vi "R1NH4Control.vi"(8 "error constant":errorcluster, 11 "LabVIEW Web Service":refnum<class "Web Service.lvclass">) -> (0 "error (out)":errorcluster)   [LabVIEW 2016]
uses:
  <vilib>/wsapi/Web Service.lvclass
  Controls/Tri State Control.ctl
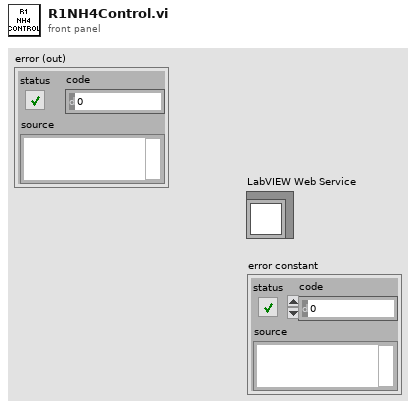
[diagram p1: front panel]
types:
  T1 = cluster{"Signal, mA":dbl, "Value, UNITS HERE":dbl}
  T2 = cluster{"Media Pump":bool, "Water Pump":bool, "Effluent Pump":bool, "Release Valve":bool, "Gas Pump":bool}
  T3 = cluster{"Set Point, mgN/L":dbl, "Tolerance, mgN/L":dbl, "Pump Gain":dbl, "Max Volume/Cycle, mL":dbl}
  T4 = typedef "Tri State Control.ctl" = u16
  T5 = cluster{"Raw Value":dbl, "Corrected Value":dbl, "Signal, mV":dbl, "Equilibrium Approach, mV/min":dbl, "Steady State?":T4}
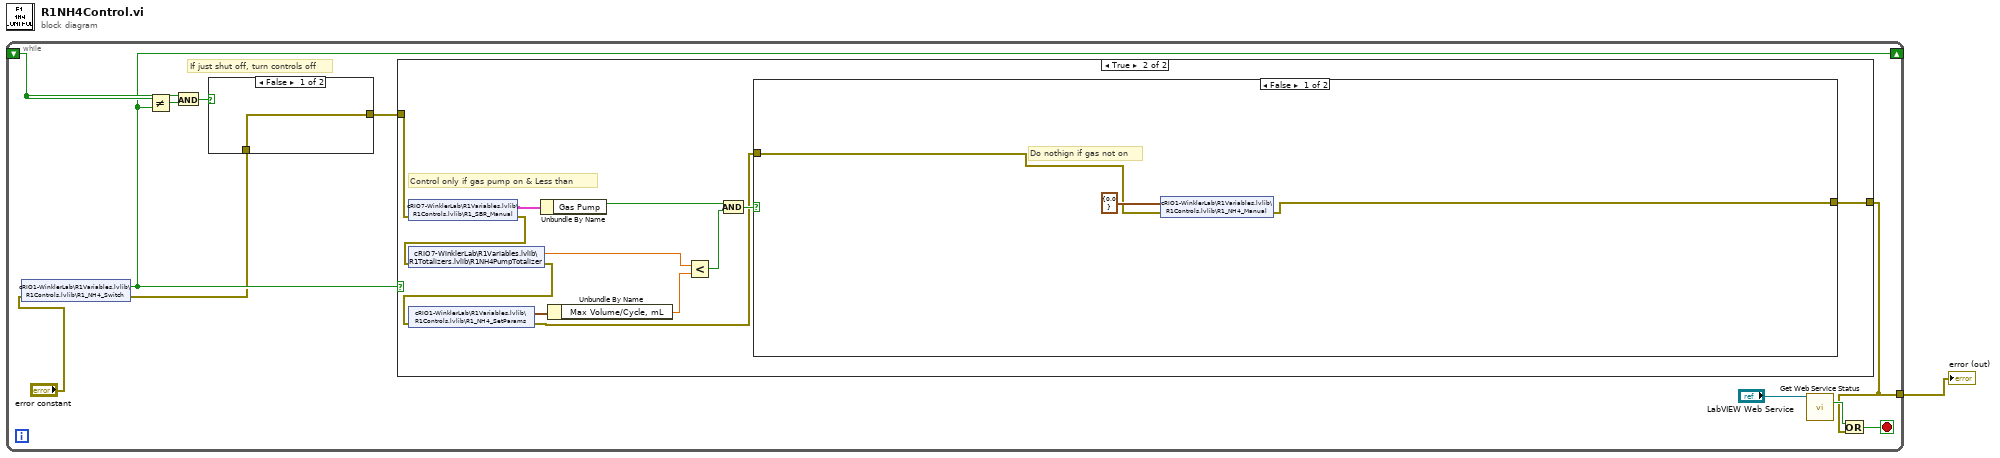
[diagram p0: block diagram]
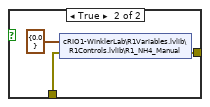
[diagram p2: hidden frame]
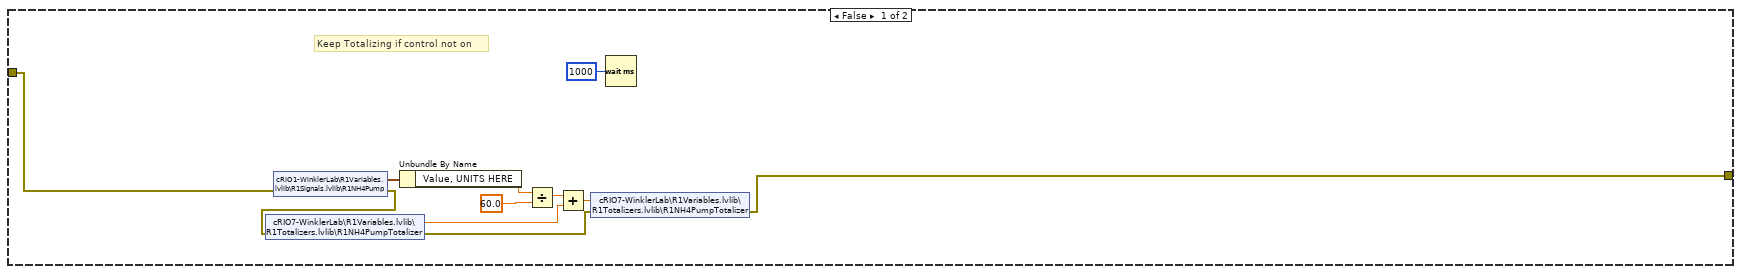
[diagram p3: hidden frame]
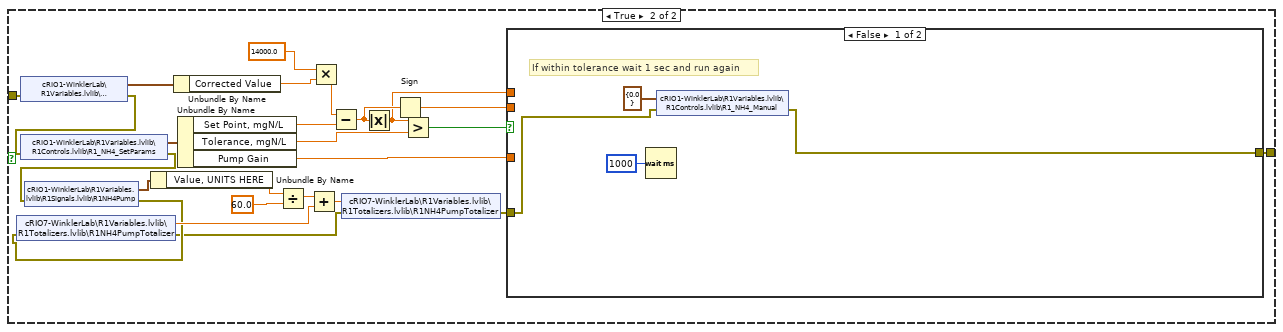
[diagram p4: hidden frame]
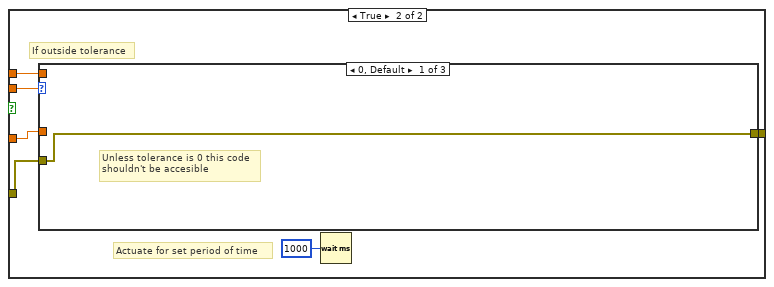
[diagram p5: hidden frame]
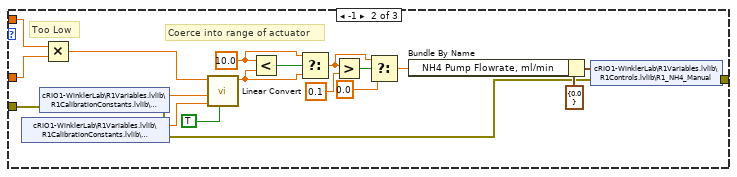
[diagram p6: hidden frame]
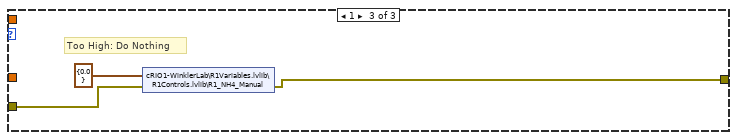
[diagram p7: hidden frame]
diagram:
  n1 = while {
    shift-right: [w6] -> _
    shift-left: _ -> [w7]
    tunnel: [w2] -> w1
    stop <- w10 stop-if-true
    # "If just shut off, turn controls off"
    n2 = shared-variable "cRIO1-WinklerLab\\R1Variables.lvlib\\R1Controls.lvlib\\R1_NH4_Switch"(error in="error constant") -> (w6:bool, error out=w5:errorcluster)
    n3 = Not Equal?(x=w7, y=w6) -> (x != y?=w8:bool)
    n4 = And(x=w7, y=w8) -> (x .and. y?=w9:bool)
    n5 = case shown="False" w9 {
      tunnel: w5 -> [w13 w15]
      tunnel: [w13 w14] -> w4
      frame False {
      }
      frame True {
        n6 = shared-variable "cRIO1-WinklerLab\\R1Variables.lvlib\\R1Controls.lvlib\\R1_NH4_Manual"(cluster{"NH4 Pump Flowrate, ml/min":dbl} {"NH4 Pump Flowrate, ml/min"=0.0} ("R1_NH4_Manual"), error in=w15) -> (error out=w14:errorcluster)
      }
    }
    n7 = case shown="True" w6 {
      tunnel: w4 -> [w20 w32]
      tunnel: [w17 w28] -> w2
      frame False {
        # "Keep Totalizing if control not on"
        n8 = shared-variable "cRIO1-WinklerLab\\R1Variables.lvlib\\R1Signals.lvlib\\R1NH4Pump"(error in=w20) -> (w22:T1, error out=w19:errorcluster)
        n9 = shared-variable "cRIO7-WinklerLab\\R1Variables.lvlib\\R1Totalizers.lvlib\\R1NH4PumpTotalizer"(error in=w19) -> (w24:dbl, error out=w18:errorcluster)
        n10 = Unbundle By Name(w22) -> ("Value, UNITS HERE"=w27:dbl)
        n11 = Divide(x=w27, y=60.0) -> (x/y=w25:dbl)
        n12 = Add(x=w25, y=w24) -> (x+y=w23:dbl)
        n13 = shared-variable "cRIO7-WinklerLab\\R1Variables.lvlib\\R1Totalizers.lvlib\\R1NH4PumpTotalizer"(w23, error in=w18) -> (error out=w17:errorcluster)
        n14 = Wait (ms)(milliseconds to wait=u32 1000) -> ()  [unwired: 1 out]
      }
      frame True {
        # "Control only if gas pump on & Less than"
        n15 = shared-variable "cRIO7-WinklerLab\\R1Variables.lvlib\\R1Controls.lvlib\\R1_SBR_Manual"(error in=w32) -> (w39:T2, error out=w31:errorcluster)
        n16 = shared-variable "cRIO7-WinklerLab\\R1Variables.lvlib\\R1Totalizers.lvlib\\R1NH4PumpTotalizer"(error in=w31) -> (w37:dbl, error out=w30:errorcluster)
        n17 = shared-variable "cRIO1-WinklerLab\\R1Variables.lvlib\\R1Controls.lvlib\\R1_NH4_SetParams"(error in=w30) -> (w38:T3, error out=w29:errorcluster)
        n18 = Unbundle By Name(w39) -> ("Gas Pump"=w34:bool)
        n19 = Unbundle By Name(w38) -> ("Max Volume/Cycle, mL"=w36:dbl)
        n20 = Less?(x=w37, y=w36) -> (x < y?=w33:bool)
        n21 = And(x=w34, y=w33) -> (x .and. y?=w35:bool)
        n22 = case shown="False" w35 {
          tunnel: w29 -> [w41 w49]
          tunnel: [w40 w43] -> w28
          frame False {
            # "Do nothign if gas not on"
            n23 = shared-variable "cRIO1-WinklerLab\\R1Variables.lvlib\\R1Controls.lvlib\\R1_NH4_Manual"(cluster{"NH4 Pump Flowrate, ml/min":dbl} {"NH4 Pump Flowrate, ml/min"=0.0} ("R1_NH4_Manual"), error in=w41) -> (error out=w40:errorcluster)
          }
          frame True {
            n24 = shared-variable "cRIO1-WinklerLab\\R1Variables.lvlib\\R1ISEVariables.lvlib\\R1_NH4_ISE"(error in=w49) -> (w60:T5, error out=w48:errorcluster)
            n25 = shared-variable "cRIO1-WinklerLab\\R1Variables.lvlib\\R1Controls.lvlib\\R1_NH4_SetParams"(error in=w48) -> (w59:T3, error out=w47:errorcluster)
            n26 = shared-variable "cRIO1-WinklerLab\\R1Variables.lvlib\\R1Signals.lvlib\\R1NH4Pump"(error in=w47) -> (w53:T1, error out=w46:errorcluster)
            n27 = shared-variable "cRIO7-WinklerLab\\R1Variables.lvlib\\R1Totalizers.lvlib\\R1NH4PumpTotalizer"(error in=w46) -> (w55:dbl, error out=w45:errorcluster)
            n28 = Unbundle By Name(w53) -> ("Value, UNITS HERE"=w58:dbl)
            n29 = Unbundle By Name(w60) -> ("Corrected Value"=w51:dbl)
            n30 = Unbundle By Name(w59) -> ("Set Point, mgN/L"=w67:dbl, "Tolerance, mgN/L"=w66:dbl, "Pump Gain"=w63:dbl)
            n31 = Divide(x=w58, y=60.0) -> (x/y=w56:dbl)
            n32 = Add(x=w56, y=w55) -> (x+y=w54:dbl)
            n33 = Multiply(x=14000.0, y=w51) -> (x*y=w50:dbl)
            n34 = Subtract(x=w50, y=w67) -> (x-y=w62:dbl)
            n35 = shared-variable "cRIO7-WinklerLab\\R1Variables.lvlib\\R1Totalizers.lvlib\\R1NH4PumpTotalizer"(w54, error in=w45) -> (error out=w44:errorcluster)
            n36 = Absolute Value(x=w62) -> (abs(x)=w61:dbl)
            n37 = Sign(1:w62) -> (0:w64:dbl)
            n38 = Greater?(x=w61, y=w66) -> (0:w65:bool)
            n39 = case shown="False" w65 {
              tunnel: w64 -> [_ w77]
              tunnel: w63 -> [_ w76]
              tunnel: w61 -> [_ w75]
              tunnel: w44 -> [w69 w73]
              tunnel: [w68 w72] -> w43
              frame False {
                # "If within tolerance wait 1 sec and run again"
                n40 = Wait (ms)(milliseconds to wait=u32 1000) -> ()  [unwired: 1 out]
                n41 = shared-variable "cRIO1-WinklerLab\\R1Variables.lvlib\\R1Controls.lvlib\\R1_NH4_Manual"(cluster{"NH4 Pump Flowrate, ml/min":dbl} {"NH4 Pump Flowrate, ml/min"=0.0} ("R1_NH4_Manual"), error in=w69) -> (error out=w68:errorcluster)
              }
              frame True {
                # "Actuate for set period of time"
                # "If outside tolerance"
                n42 = case shown="0, Default" w77 {
                  tunnel: w76 -> [_ w97 _]
                  tunnel: w75 -> [_ w98 _]
                  tunnel: w73 -> [w78 w82 w100]
                  tunnel: [w78 w79 w99] -> w72
                  frame 0, Default {
                    # "Unless tolerance is 0 this code\nshouldn't be accesible"
                  }
                  frame -1 {
                    w91 = 10.0
                    # "Coerce into range of actuator"
                    # "Too Low"
                    n43 = shared-variable "cRIO1-WinklerLab\\R1Variables.lvlib\\R1CalibrationConstants.lvlib\\NH4PumpSlope"(error in=w82) -> (w94:dbl, error out=w81:errorcluster)
                    n44 = shared-variable "cRIO1-WinklerLab\\R1Variables.lvlib\\R1CalibrationConstants.lvlib\\NH4PumpIntercept"(error in=w81) -> (w93:dbl, error out=w80:errorcluster)
                    n45 = Multiply(x=w98, y=w97) -> (x*y=w85:dbl)
                    n46 = call "Linear Convert.vi"("Inverse?"=TRUE, "Intercept"=w93, "Slope"=w94, "Signal"=w85) -> ("Result"=w89:dbl)  [unwired: 7 in]
                    n47 = Less?(x=w91, y=w89) -> (x < y?=w90:bool)
                    n48 = Select(t=w91, s=w90, f=w89) -> (s? t:f=w87:dbl)
                    n49 = Greater?(x=w87, y=0.1) -> (0:w88:bool)
                    n50 = Select(t=w87, s=w88, f=0.0) -> (s? t:f=w84:dbl)
                    n51 = Bundle By Name(cluster=cluster{"NH4 Pump Flowrate, ml/min":dbl} {"NH4 Pump Flowrate, ml/min"=0.0} ("R1_NH4_Manual"), "NH4 Pump Flowrate, ml/min"=w84) -> (w96:cluster{"NH4 Pump Flowrate, ml/min":dbl})
                    n52 = shared-variable "cRIO1-WinklerLab\\R1Variables.lvlib\\R1Controls.lvlib\\R1_NH4_Manual"(w96, error in=w80) -> (error out=w79:errorcluster)
                  }
                  frame 1 {
                    # "Too High: Do Nothing"
                    n53 = shared-variable "cRIO1-WinklerLab\\R1Variables.lvlib\\R1Controls.lvlib\\R1_NH4_Manual"(cluster{"NH4 Pump Flowrate, ml/min":dbl} {"NH4 Pump Flowrate, ml/min"=0.0} ("R1_NH4_Manual"), error in=w100) -> (error out=w99:errorcluster)
                  }
                }
                n54 = Wait (ms)(milliseconds to wait=u32 1000) -> ()  [unwired: 1 out]
              }
            }
          }
        }
      }
    }
    n55 = call <vilib>:"Get Web Service Status.vi"("LabVIEW Web Service"="LabVIEW Web Service") -> ("service stopping?"=w12:bool)  [unwired: 12 in, 2 out]
    n56 = Or(x=w12, y=w2) -> (x .or. y?=w10:bool)
  }
  "error (out)" <- w1
